vi "IMU_Ref_Num.vi"() -> (3 "IMU_Reft_Num":T1={"DevStatus"={"status"=FALSE, "code"=0, "source"=""}, "Gyro Address"=0, "Gyro Range"=0, "Mean Rates"={"Xmo"=0.0, "Ymo"=0.0, "Zmo"=0.0}, "StdDev Rates"={"Xsdo"=0.0, "Ysdo"=0.0, "Zsdo"=0.0}, "Fast"=FALSE, "Reset"=FALSE, "Accel Address"=0, "Accel Range"=0, "Accel Scale"={"Xscale"=0.0, "Yscale"=0.0, "Zscale"=0.0}, "Mag Address"=0, "Mag Range"=0, "G Sense"=FALSE, "A Sense"=FALSE, "M Sense"=FALSE, "Accel Offset"={"Xzero"=0.0, "Yzero"=0.0, "Zzero"=0.0}, "Motion Thresh"=0.0, "Mag Scale"={"Xscale"=1.0, "Yscale"=1.0, "Zscale"=1.0}, "Mag Offset"={"Xzero"=1.0, "Yzero"=1.0, "Zzero"=1.0}, "I2C Bus"=enum."I2C On-Board", "Handle"=0, "Controller"=enum."Controller 1", "Anomaly Thresh"=0.0, "Local Mag"=0.0})   [LabVIEW 2014]
uses:
  AdaIMU roboRIO/IMUDevRef.ctl
  <vilib>/Rock Robotics/SystemInterfaces/i2clib/i2c_bus.ctl
  <vilib>/Rock Robotics/SystemInterfaces/Typedef/FPGA_TypedefDigitalModule.ctl
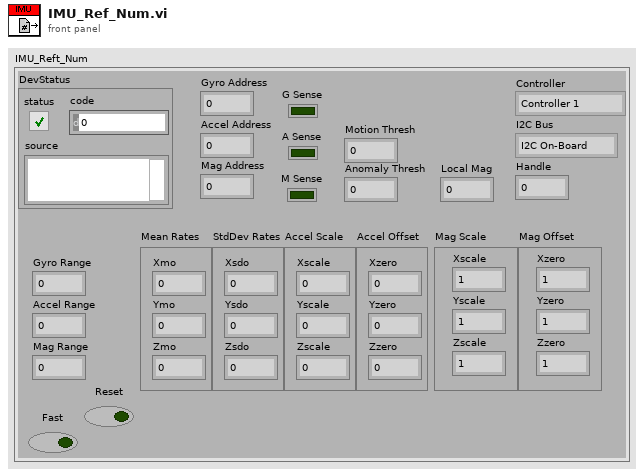
[diagram p1: front panel]
types:
  T1 = typedef "IMUDevRef.ctl" = cluster{"DevStatus":errorcluster, "Gyro Address":u8, "Gyro Range":u8, "Mean Rates":cluster{"Xmo":dbl, "Ymo":dbl, "Zmo":dbl}, "StdDev Rates":cluster{"Xsdo":dbl, "Ysdo":dbl, "Zsdo":dbl}, "Fast":bool, "Reset":bool, "Accel Address":u8, "Accel Range":u8, "Accel Scale":cluster{"Xscale":dbl, "Yscale":dbl, "Zscale":dbl}, "Mag Address":u8, "Mag Range":u8, "G Sense":bool, "A Sense":bool, "M Sense":bool, "Accel Offset":cluster{"Xzero":dbl, "Yzero":dbl, "Zzero":dbl}, "Motion Thresh":dbl, "Mag Scale":cluster{"Xscale":dbl, "Yscale":dbl, "Zscale":dbl}, "Mag Offset":cluster{"Xzero":dbl, "Yzero":dbl, "Zzero":dbl}, "I2C Bus":T2, "Handle":i32, "Controller":T3, "Anomaly Thresh":dbl, "Local Mag":dbl}
  T2 = typedef "i2c_bus.ctl" = enum16{"I2C On-Board", "I2C MXP", "Invalid"}
  T3 = typedef "FPGA_TypedefDigitalModule.ctl" = enum16{"Controller 1"}
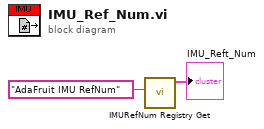
[diagram p0: block diagram]
diagram:
  n1 = call "IMURefNum Registry Get.vi"("refnum name"="AdaFruit IMU RefNum") -> ("AdaIMUDevRef Out"=→"IMU_Reft_Num":T1)  [unwired: 9 in, 1 out]
